vi "top_set_measurement_type_specifics.vi"(11 "Input parameters":T1={"Measurement type"=enum."Debug", "Sensor type"=enum."IFX_8in_256ch", "Identifier"="test.txt", "Open after execution?"=FALSE, "Plot after execution?"=FALSE, "Display channel"=0, "Voltage Delay (s)"=0.5, "Switch Delay (s)"=0.01, "VISA resource name source"="", "VISA resource name DMM"="", "VISA resource name LCR"="", "Compliance  Level (A)"=1e-05, "Voltage Limit (V)"=1000.0, "Data storage location"="", "Scan voltages"="", "Use source as DMM?"=FALSE, "LCR signal frequenzy (Hz)"=10000.0, "DMM device"=enum."Keithley2450", "Sampling number"=1, "Use env. sensors on"=enum."Sensirion sht1x/7x", "Switchboard Handle"=0, "Use Switchboard"=FALSE, "LCR signal voltage (V)"=10000.0, "Repeat"=1, "Scan voltages IV"="", "Scan voltages CV"="", "Hex pad numbers?"=FALSE, "Set measurement type"=enum."Debug", "Custom pad scan"="", "IV voltage Delay (s)"=0.5, "CV voltage Delay (s)"=0.5, "Needle measurement?"=FALSE, "Comments"="test.txt", "LCR signal frequenzy (kHz)"=10.0, "Compliance  Level (uA)"=10.0, "Open Correction Array"=array2304x3[6912 elements], "Current set voltage"=0.0, "Last set voltage"=0.0, "Current channel"=0, "Last OpenCorrection index"=-1, "Total curr/vltg every x steps"=10, "Current channel iteration"=0, "No CV corrections"=FALSE, "Mapfile"="", "Corrfile"="", "IV voltage file"=path "", "CV voltage file"=path "", "IV Switch Delay (s)"=0.01, "CV Switch Delay (s)"=0.01, "Invert polarity"=FALSE, "Set debug dirs"=FALSE, "Is n on p"=FALSE, "Source interlock?"=TRUE, "Voltage file used?"=FALSE, "Pad mask"=""} {"CV Switch Delay (s)" format="%#_13g"; "IV Switch Delay (s)" format="%#_13g"; "Last set voltage" format="%#_13g"; "Current set voltage" format="%#_13g"; "CV voltage Delay (s)" format="%#_13g"; "IV voltage Delay (s)" format="%#_13g"; "Voltage Limit (V)" format="%#_13g"; "Voltage Delay (s)" format="%#_13g"; "Switch Delay (s)" format="%#_13g"}) -> (3 "Input parameters out":T1={"Measurement type"=enum."Debug", "Sensor type"=enum."IFX_8in_256ch", "Identifier"="test.txt", "Open after execution?"=FALSE, "Plot after execution?"=FALSE, "Display channel"=0, "Voltage Delay (s)"=0.5, "Switch Delay (s)"=0.01, "VISA resource name source"="", "VISA resource name DMM"="", "VISA resource name LCR"="", "Compliance  Level (A)"=1e-05, "Voltage Limit (V)"=1000.0, "Data storage location"="", "Scan voltages"="", "Use source as DMM?"=FALSE, "LCR signal frequenzy (Hz)"=10000.0, "DMM device"=enum."Keithley2450", "Sampling number"=1, "Use env. sensors on"=enum."Sensirion sht1x/7x", "Switchboard Handle"=0, "Use Switchboard"=FALSE, "LCR signal voltage (V)"=10000.0, "Repeat"=1, "Scan voltages IV"="", "Scan voltages CV"="", "Hex pad numbers?"=FALSE, "Set measurement type"=enum."Debug", "Custom pad scan"="", "IV voltage Delay (s)"=0.5, "CV voltage Delay (s)"=0.5, "Needle measurement?"=FALSE, "Comments"="test.txt", "LCR signal frequenzy (kHz)"=10.0, "Compliance  Level (uA)"=10.0, "Open Correction Array"=array2304x3[6912 elements], "Current set voltage"=0.0, "Last set voltage"=0.0, "Current channel"=0, "Last OpenCorrection index"=-1, "Total curr/vltg every x steps"=10, "Current channel iteration"=0, "No CV corrections"=FALSE, "Mapfile"="", "Corrfile"="", "IV voltage file"=path "", "CV voltage file"=path "", "IV Switch Delay (s)"=0.01, "CV Switch Delay (s)"=0.01, "Invert polarity"=FALSE, "Set debug dirs"=FALSE, "Is n on p"=FALSE, "Source interlock?"=TRUE, "Voltage file used?"=FALSE, "Pad mask"=""} {"CV Switch Delay (s)" format="%#_13g"; "IV Switch Delay (s)" format="%#_13g"; "Last set voltage" format="%#_13g"; "Current set voltage" format="%#_13g"; "CV voltage Delay (s)" format="%#_13g"; "IV voltage Delay (s)" format="%#_13g"; "Voltage Limit (V)" format="%#_13g"; "Voltage Delay (s)" format="%#_13g"; "Switch Delay (s)" format="%#_13g"})   [LabVIEW 2016]
doc: "Set IV/CV dependent voltages, units and names."
uses:
  input_params.ctl
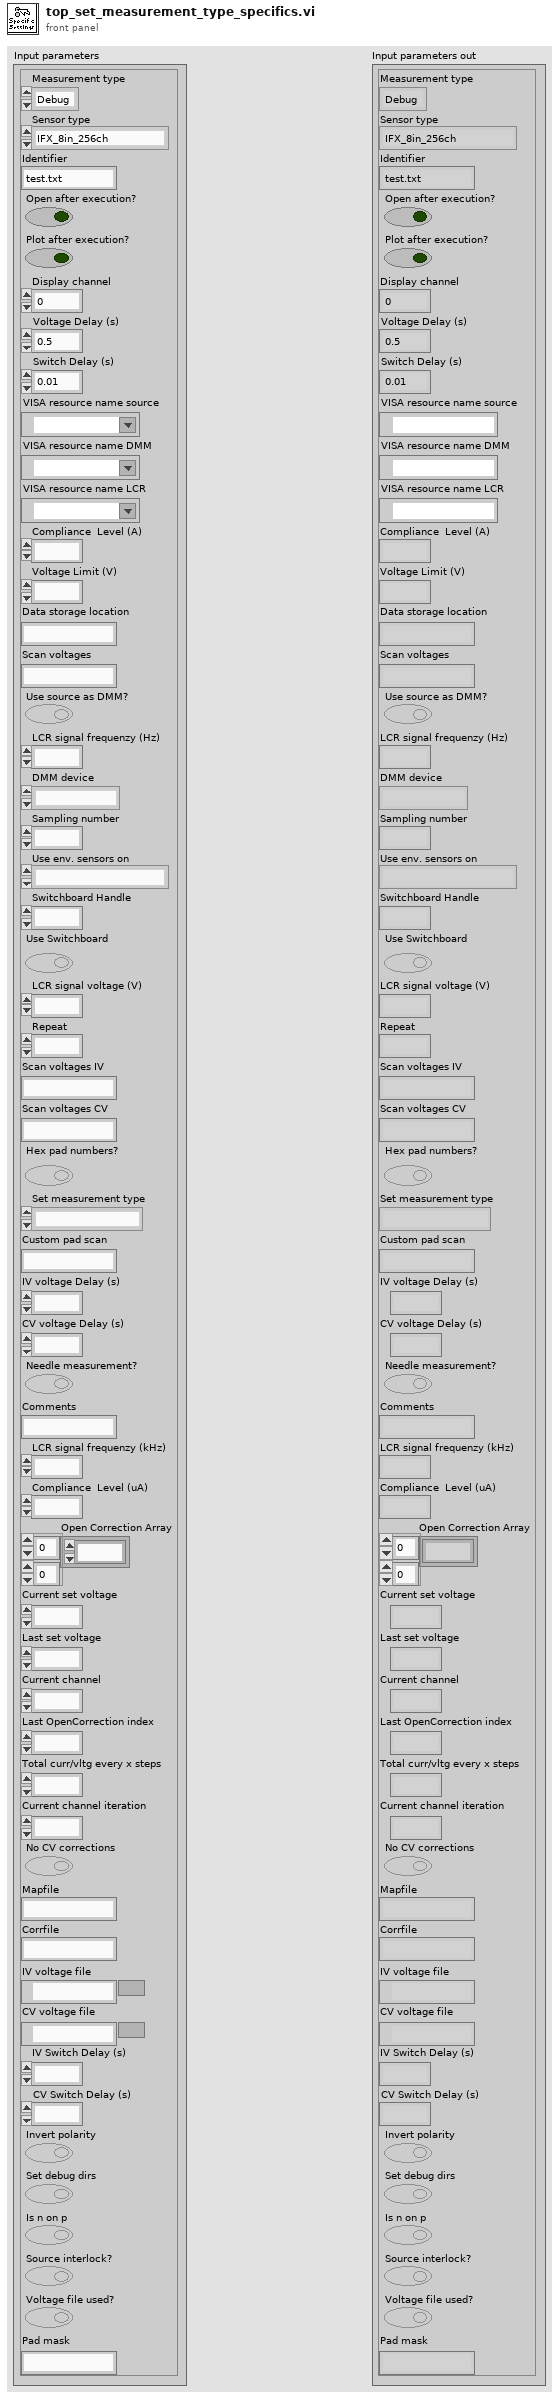
[diagram p1: front panel]
types:
  T1 = typedef "input_params.ctl" = cluster{"Measurement type":enum16{"IV", "CV", "Debug", "Test_contact"}, "Sensor type":enum16{"HPK_6in_135ch", "HPK_8in_271ch", "IFX_8in_256ch", "Diode", "HPK_6in_239ch", "Full_Matrix", ""}, "Identifier":string, "Open after execution?":bool, "Plot after execution?":bool, "Display channel":i32, "Voltage Delay (s)":dbl, "Switch Delay (s)":dbl, "VISA resource name source":refnum<visa-resource-name>, "VISA resource name DMM":refnum<visa-resource-name>, "VISA resource name LCR":refnum<visa-resource-name>, "Compliance  Level (A)":dbl, "Voltage Limit (V)":dbl, "Data storage location":string, "Scan voltages":string, "Use source as DMM?":bool, "LCR signal frequenzy (Hz)":dbl, "DMM device":enum16{"Keithley2001", "Keithley2450", "Keithley2410", "Keithley6487", "Keithley6517"}, "Sampling number":i32, "Use env. sensors on":enum16{"Sensirion sht1x/7x", "Switch Matrix", "Probecard"}, "Switchboard Handle":u32, "Use Switchboard":bool, "LCR signal voltage (V)":dbl, "Repeat":i32, "Scan voltages IV":string, "Scan voltages CV":string, "Hex pad numbers?":bool, "Set measurement type":enum16{"IV", "CV", "Debug", "Test_contact", "IV+CV"}, "Custom pad scan":string, "IV voltage Delay (s)":dbl, "CV voltage Delay (s)":dbl, "Needle measurement?":bool, "Comments":string, "LCR signal frequenzy (kHz)":dbl, "Compliance  Level (uA)":dbl, "Open Correction Array":dbl[][], "Current set voltage":dbl, "Last set voltage":dbl, "Current channel":i32, "Last OpenCorrection index":i32, "Total curr/vltg every x steps":i32, "Current channel iteration":i32, "No CV corrections":bool, "Mapfile":string, "Corrfile":string, "IV voltage file":path, "CV voltage file":path, "IV Switch Delay (s)":dbl, "CV Switch Delay (s)":dbl, "Invert polarity":bool, "Set debug dirs":bool, "Is n on p":bool, "Source interlock?":bool, "Voltage file used?":bool, "Pad mask":string}
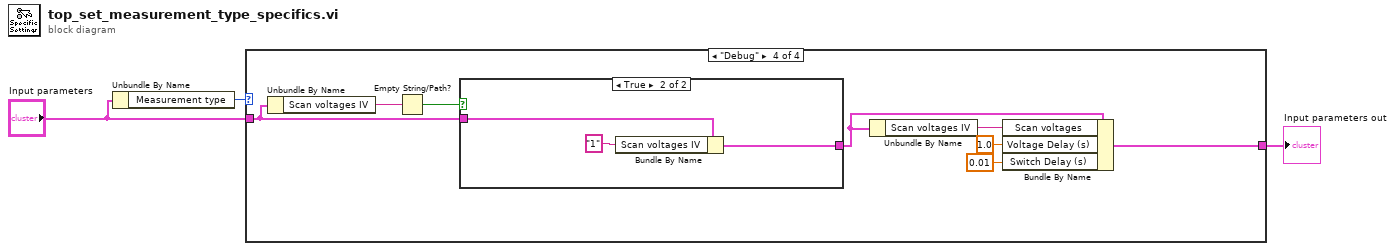
[diagram p0: block diagram]
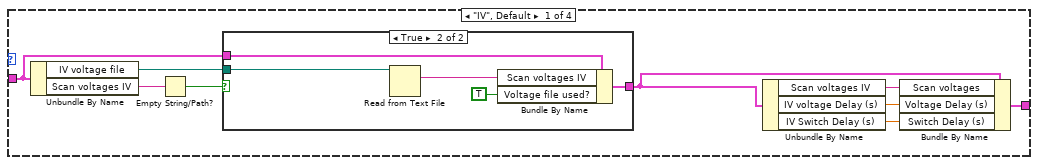
[diagram p2: hidden frame]
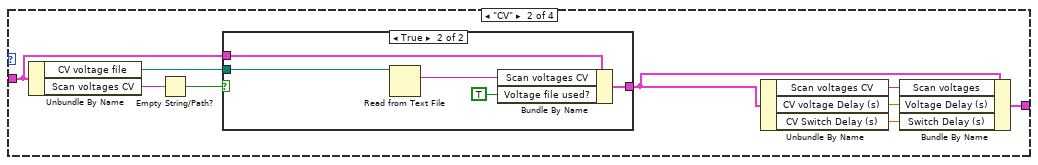
[diagram p4: hidden frame]
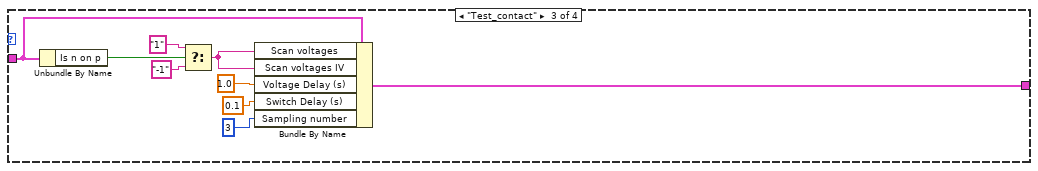
[diagram p6: hidden frame]
diagram:
  n1 = Unbundle By Name("Input parameters") -> ("Measurement type"=w3:enum16{"IV", "CV", "Debug", "Test_contact"})
  n2 = case shown="\"Debug\"" w3 {
    tunnel: "Input parameters" -> [w5 w20 w38 w46]
    tunnel: [w11 w27 w42 w45] -> w1
    frame "IV", Default {
      n3 = Unbundle By Name(w5) -> ("IV voltage file"=w8:path, "Scan voltages IV"=w7:string)
      n4 = Empty String/Path?(string/path=w7) -> (empty?=w6:bool)
      n5 = case shown="True" w6 {
        tunnel: [w13 w17] -> w4
        tunnel: w8 -> [_ w18]
        tunnel: w5 -> [w13 w15]
        frame False {
        }
        frame True {
          n6 = Read from Text File(file (use dialog)=w18) -> (text=w16:string)  [unwired: 3 in, 3 out]
          n7 = Bundle By Name(cluster=w15, "Scan voltages IV"=w16, "Voltage file used?"=TRUE) -> (w17:T1)
        }
      }
      n8 = Unbundle By Name(w4) -> ("Scan voltages IV"=w12:string, "IV voltage Delay (s)"=w10:dbl, "IV Switch Delay (s)"=w9:dbl)
      n9 = Bundle By Name(cluster=w4, "Scan voltages"=w12, "Voltage Delay (s)"=w10, "Switch Delay (s)"=w9) -> (w11:T1)
    }
    frame "CV" {
      n10 = Unbundle By Name(w20) -> ("CV voltage file"=w21:path, "Scan voltages CV"=w22:string)
      n11 = Empty String/Path?(string/path=w22) -> (empty?=w23:bool)
      n12 = case shown="True" w23 {
        tunnel: [w28 w32] -> w19
        tunnel: w21 -> [_ w33]
        tunnel: w20 -> [w28 w30]
        frame False {
        }
        frame True {
          n13 = Read from Text File(file (use dialog)=w33) -> (text=w31:string)  [unwired: 3 in, 3 out]
          n14 = Bundle By Name(cluster=w30, "Scan voltages CV"=w31, "Voltage file used?"=TRUE) -> (w32:T1)
        }
      }
      n15 = Unbundle By Name(w19) -> ("Scan voltages CV"=w26:string, "CV voltage Delay (s)"=w25:dbl, "CV Switch Delay (s)"=w24:dbl)
      n16 = Bundle By Name(cluster=w19, "Scan voltages"=w26, "Voltage Delay (s)"=w25, "Switch Delay (s)"=w24) -> (w27:T1)
    }
    frame "Test_contact" {
      n17 = Unbundle By Name(w38) -> ("Is n on p"=w37:bool)
      n18 = Select(t="1" ("Scan voltages"), s=w37, f="-1" ("Scan voltages")) -> (s? t:f=w34:string)
      n19 = Bundle By Name(cluster=w38, "Scan voltages"=w34, "Scan voltages IV"=w34, "Voltage Delay (s)"=1.0, "Switch Delay (s)"=0.1, "Sampling number"=3) -> (w42:T1)
    }
    frame "Debug" {
      n20 = Unbundle By Name(w46) -> ("Scan voltages IV"=w49:string)
      n21 = Empty String/Path?(string/path=w49) -> (empty?=w48:bool)
      n22 = case shown="True" w48 {
        tunnel: [w51 w54] -> w47
        tunnel: w46 -> [w51 w53]
        frame False {
        }
        frame True {
          n23 = Bundle By Name(cluster=w53, "Scan voltages IV"="1") -> (w54:T1)
        }
      }
      n24 = Unbundle By Name(w47) -> ("Scan voltages IV"=w50:string)
      n25 = Bundle By Name(cluster=w47, "Scan voltages"=w50, "Voltage Delay (s)"=1.0, "Switch Delay (s)"=0.01) -> (w45:T1)
    }
  }
  "Input parameters out" <- w1
